vi "Read VacuumLine Params.vi"(8 "error in (no error)":errorcluster, 11 "VacuumLine in":refnum<class "VacuumLine.lvclass">) -> (0 "error out":errorcluster, 2 "Position Params":T1 {"max( |Motor Pos - LRF Distance| )" min=0.0}, 3 "VacuumLine out":refnum<class "VacuumLine.lvclass">)   [LabVIEW 2016, in "Hardware.lvlib" / "VacuumLine.lvlib" / "VacuumLine.lvclass"]
uses:
  <userlib>/Common Components/Hardware/Abstract System/VacuumLine/VacuumLine/VacuumLine.lvclass
  <userlib>/Common Components/Hardware/Abstract System/VacuumLine/VacuumLine/VacuumLine Params.ctl
  <userlib>/Common Components/Hardware/Abstract System/VacuumLine/VacuumLine/Valve Complex.ctl
  <userlib>/Common Components/Hardware/Abstract System/VacuumLine/VacuumLine/Logic Cluster.ctl
  <userlib>/Common Components/Hardware/Abstract System/VacuumLine/VacuumLine/VacuumLine.lvclass/VacuumLine.ctl
panel:
  # "Pin#"
  # "Location"
  # "Tolerance"
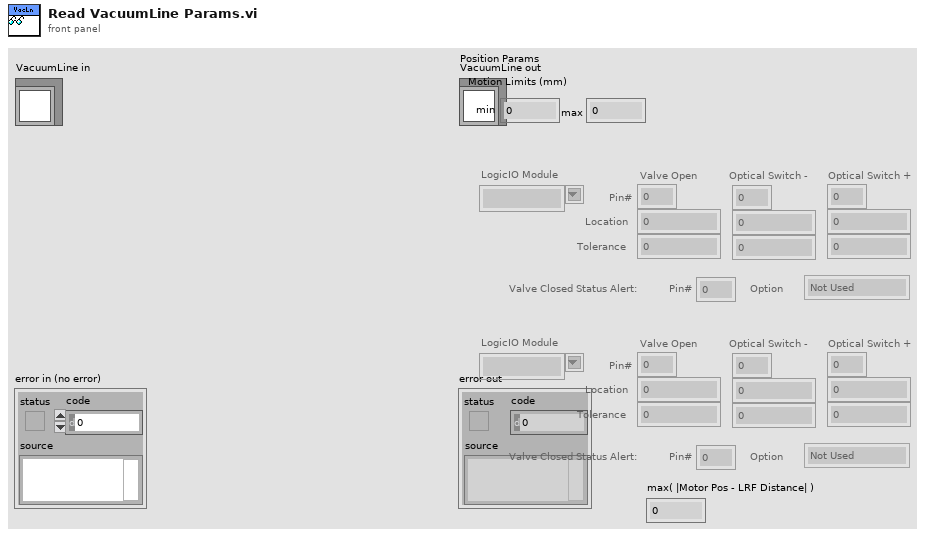
[diagram p1: front panel]
types:
  T1 = typedef "Hardware.lvlib/VacuumLine.lvlib/VacuumLine.lvclass/VacuumLine Params.ctl" = cluster{"Motion Limits":cluster{"min":dbl, "max":dbl}, "Valve Complexes":T2[], "max( |Motor Pos - LRF Distance| )":dbl}
  T2 = typedef "Hardware.lvlib/VacuumLine.lvlib/VacuumLine.lvclass/Valve Complex.ctl" = cluster{"LogicIO Module":string, "Valve Open":T3, "Optical Switch -":T3, "Optical Switch +":T3, "Valve Closed Status Alert":cluster{"Pin#":u8, "Option":enum16{"Not Used", "Normally Closed"}}}
  T3 = typedef "Hardware.lvlib/VacuumLine.lvlib/VacuumLine.lvclass/Logic Cluster.ctl" = cluster{"Pin#":u8, "Location":dbl, "Tolerance":dbl}
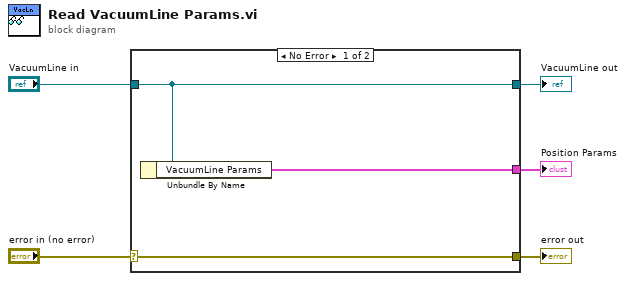
[diagram p0: block diagram]
diagram:
  n1 = case shown="No Error" "error in (no error)" {
    selector: "error in (no error)" -> [w8 w9]
    tunnel: [w8 w9] -> w4
    tunnel: [w7 w10] -> w2
    tunnel: "VacuumLine in" -> [w7 w10]
    tunnel: [w6 _] -> w1
    frame No Error {
      n2 = Unbundle By Name(w7) -> ("VacuumLine Params"=w6:T1)
    }
    frame Error {
    }
  }
  "error out" <- w4
  "VacuumLine out" <- w2
  "Position Params" <- w1
